vi "Problem1.9-RandomNumbers.vi"() -> ()   [LabVIEW 2019]
panel:
  out "Min Index":i32[](array[numeric])
  out "Max Index":i32[](array[numeric])
  out "Min Value":dbl
  out "Max Value":dbl
  out "Array Size":i32[](array[numeric])
  out "Original Random Number Array":dbl[][](array[numeric])
  out "Uniform Deviates Array":dbl[][](array[numeric])
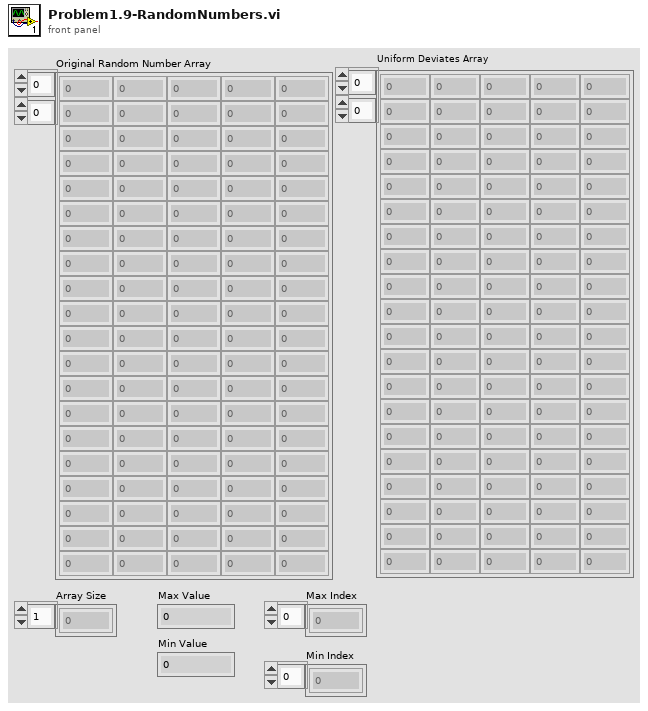
[diagram p1: front panel]
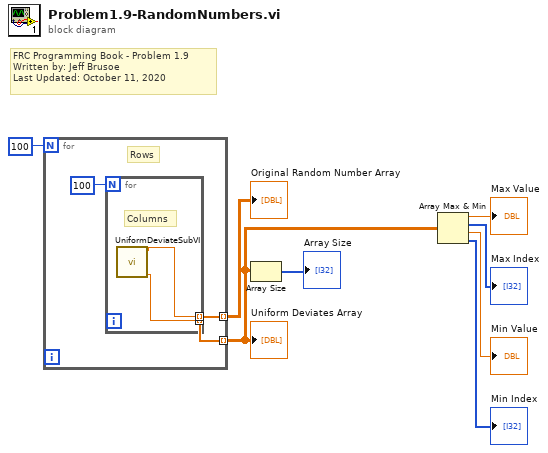
[diagram p0: block diagram]
diagram:
  # "FRC Programming Book - Problem 1.9\nWritten by: Jeff Brusoe\nLast Updated: October 11, 2020"
  n1 = for {
    N: 100 -> [_]
    tunnel: [w10] -> w5 mode=indexing
    tunnel: [w9] -> w7 mode=indexing
    # "Rows"
    n2 = for {
      N: 100 -> [_]
      tunnel: [w12] -> w10 mode=indexing
      tunnel: [w13] -> w9 mode=indexing
      # "Columns"
      n3 = call "UniformDeviateSubVI.vi"() -> ("Uniform Deviate"=w12:dbl, "Initial Random Number"=w13:dbl)  [unwired: 10 in]
    }
  }
  "Uniform Deviates Array" <- w5
  "Original Random Number Array" <- w7
  n4 = Array Size(array=w5) -> (size(s)=→"Array Size":i32[])
  n5 = Array Max & Min(array=w5) -> (max value=→"Max Value":dbl, max index (indices)=→"Max Index":i32[], min value=→"Min Value":dbl, min index (indices)=→"Min Index":i32[])
